vi "organize repeating list.vi"(1 "Array in":i16[](array[numeric])) -> (0 "Array out":cluster{i16, i32[]}[](array[cluster]))   [LabVIEW 2009]
panel:
  in  "estimated # of occurances":sgl=3.0
  in  "STOP":bool
  out "progress 2":u16(slide) scale=0.0..138.0
  out "progress 1":u16(slide) scale=0.0..6717.33349609375
  # "progress"
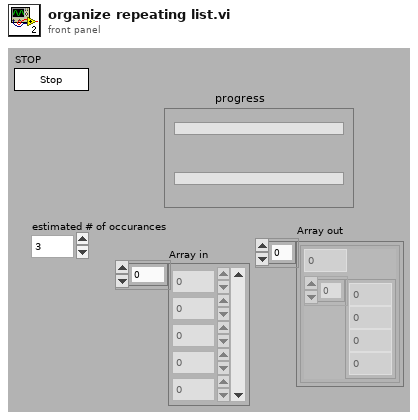
[diagram p1: front panel]
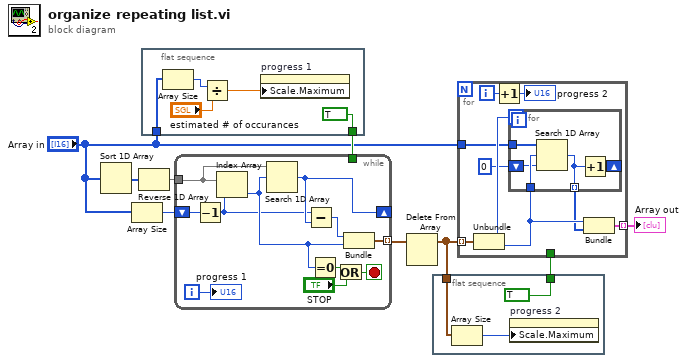
[diagram p0: block diagram]
diagram:
  n1 = Sort 1D Array(array="Array in") -> (sorted array=w9:i16[])
  n2 = Array Size(array="Array in") -> (size(s)=w4:i32)
  n3 = Reverse 1D Array(array=w9) -> (reversed array=w8:i16[])
  n4 = flat-sequence {
    tunnel: "Array in" -> [w14]
    tunnel: [TRUE] -> w5
    frame #0 {
      n5 = Array Size(array=w14) -> (size(s)=w12:i32)
      n6 = Divide(x=w12, y="estimated # of occurances") -> (x/y=w10:sgl)
      n7 = property on="progress 1" class="Slide (strict)"("Scale.Maximum"=w10) -> ()  [unwired: 2 in, 2 out]
    }
  }
  n8 = while {
    tunnel: w8 -> [w25]
    shift-right: [w16] -> _
    shift-left: w4 -> [w24]
    tunnel: [w23] -> w7 mode=indexing
    tunnel: w5 -> [_]
    i -> [w21]
    stop <- w19 stop-if-true
    n9 = Decrement(x=w24) -> (x-1=w15:i32)
    n10 = Index Array(array=w25, index=w15) -> (element=w18:i16)
    n11 = Search 1D Array(1D array=w25, element=w18) -> (index of element=w16:i32)  [unwired: 1 in]
    n12 = Subtract(x=w15, y=w16) -> (x-y=w22:i32)
    n13 = Equal To 0?(x=w18) -> (x = 0?=w20:bool)
    n14 = Or(x=w20, y="STOP") -> (x .or. y?=w19:bool)
    n15 = Bundle(w22, w18) -> (w23:cluster{i32, i16})  [unwired: 1 in]
    "progress 1" <- w21
  }
  n16 = Delete From Array(array=w7) -> (array with subset deleted=w2:cluster{i32, i16}[])  [unwired: 2 in, 1 out]
  n17 = flat-sequence {
    tunnel: w2 -> [w28]
    tunnel: [TRUE] -> w6
    frame #0 {
      n18 = Array Size(array=w28) -> (size(s)=w26:i32)
      n19 = property on="progress 2" class="Slide (strict)"("Scale.Maximum"=w26) -> ()  [unwired: 2 in, 2 out]
    }
  }
  n20 = for {
    tunnel: w2 -> [w37] mode=indexing
    tunnel: "Array in" -> [w35]
    tunnel: [w32] -> w1 mode=indexing
    tunnel: w6 -> [_]
    i -> [w31]
    n21 = Unbundle(w37) -> (w36:i32, w34:i16)
    n22 = Increment(x=w31) -> (x+1=→"progress 2":i32)
    n23 = for {
      N: w36 -> [_]
      tunnel: w34 -> [w41]
      shift-right: [w38] -> _
      shift-left: 0 -> [w40]
      tunnel: w35 -> [w42]
      tunnel: [w39] -> w33 mode=indexing
      n24 = Search 1D Array(1D array=w42, element=w41, start index (0)=w40) -> (index of element=w39:i32)
      n25 = Increment(x=w39) -> (x+1=w38:i32)
    }
    n26 = Bundle(w34, w33) -> (w32:cluster{i16, i32[]})  [unwired: 1 in]
  }
  "Array out" <- w1
